vi "Read Hardware.lvlib_CCD monitor.lvlib_CCD monitor.lvclass.vi"(8 "error in (no error)":errorcluster, 11 "CCD monitor configuration in":refnum<class "CCD monitor configuration.lvclass">) -> (0 "error out":errorcluster, 2 "Hardware.lvlib:CCD monitor.lvlib:CCD monitor.lvclass":refnum<class "CCD monitor.lvclass">, 3 "CCD monitor configuration out":refnum<class "CCD monitor configuration.lvclass">)   [LabVIEW 2016, in "CCD monitor.lvlib" / "CCD monitor configuration.lvclass"]
uses:
  <userlib>/Common Components/Hardware/Abstract System/Monitor/CCD monitor configuration.lvclass
  <userlib>/Common Components/Hardware/Abstract System/Monitor/CCD monitor.lvclass
  <userlib>/Common Components/Hardware/Abstract System/Monitor/CCD monitor configuration.lvclass/CCD monitor configuration.ctl
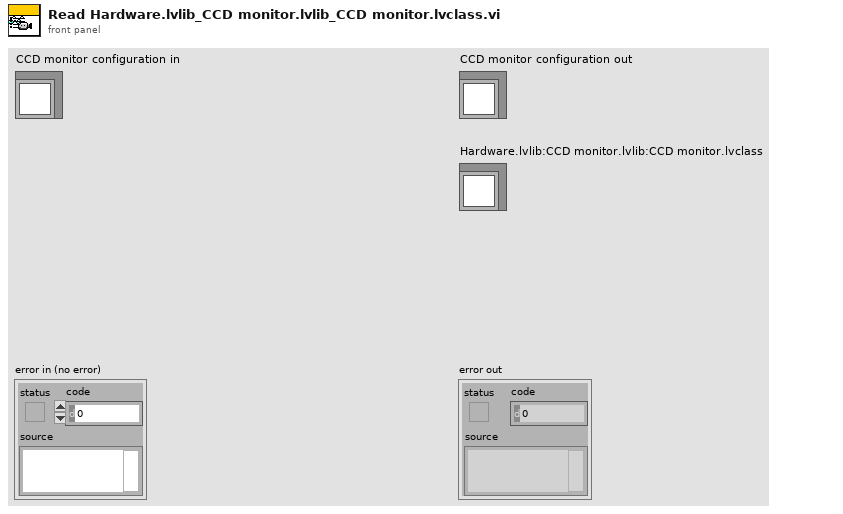
[diagram p1: front panel]
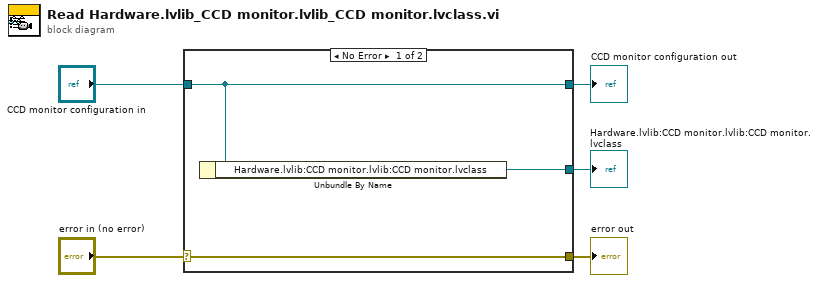
[diagram p0: block diagram]
diagram:
  n1 = case shown="No Error" "error in (no error)" {
    selector: "error in (no error)" -> [w8 w9]
    tunnel: [w8 w9] -> w4
    tunnel: [w7 w10] -> w2
    tunnel: "CCD monitor configuration in" -> [w7 w10]
    tunnel: [w6 _] -> w1
    frame No Error {
      n2 = Unbundle By Name(w7) -> ("Hardware.lvlib:CCD monitor.lvlib:CCD monitor.lvclass"=w6:refnum<class "CCD monitor.lvclass">)
    }
    frame Error {
    }
  }
  "error out" <- w4
  "CCD monitor configuration out" <- w2
  "Hardware.lvlib:CCD monitor.lvlib:CCD monitor.lvclass" <- w1
